vi "Generate Border User Layer.vi"(10 "color(black)":u32(colorbox)) -> (3 "User Layer data":T1)   [LabVIEW 2020, in "LabVIEW Icon API.lvlib"]
doc: "Generate a default Border Image Data glyph."
uses:
  <vilib>/LabVIEW Icon API/LabVIEW Icon API.lvlib
  <vilib>/LabVIEW Icon API/API_User Layer Data.ctl
  <vilib>/Utility/miscctls.llb/LVPoint32TypeDef.ctl
  <vilib>/picture/picture.llb/imagedata.ctl
panel:
  in  "Border":string="Border"
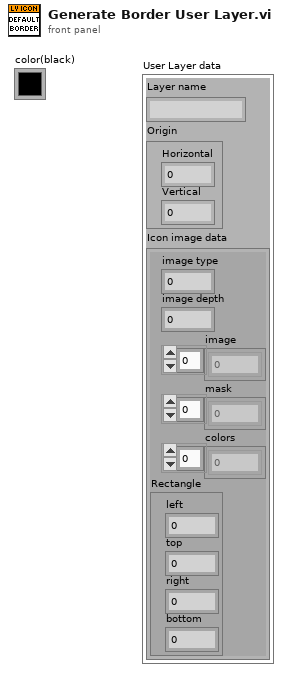
[diagram p1: front panel]
types:
  T1 = typedef "LabVIEW Icon API.lvlib/API_User Layer Data.ctl" = cluster{"Layer name":string, "Origin":T2, "Icon image data":T3}
  T2 = typedef "LVPoint32TypeDef.ctl" = cluster{"Horizontal":i32, "Vertical":i32}
  T3 = typedef "imagedata.ctl" = cluster{"image type":i32, "image depth":i32, "image":u8[], "mask":u8[], "colors":u32[], "Rectangle":cluster{"left":i16, "top":i16, "right":i16, "bottom":i16}}
  T4 = cluster{"left":i16, "top":i16, "right":i16, "bottom":i16}
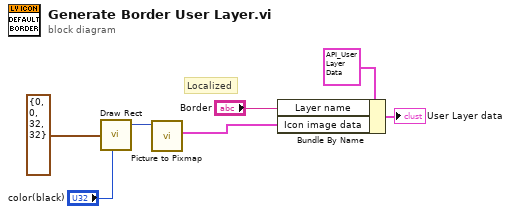
[diagram p0: block diagram]
diagram:
  # "Localized"
  n1 = call <vilib>:"Draw Rect.vi"("rect"=T4 {"left"=0, "top"=0, "right"=32, "bottom"=32}, "color(black)"="color(black)") -> ("new picture"=w2:picture)  [unwired: 7 in]
  n2 = call <vilib>:"Picture to Pixmap.vi"("picture"=w2) -> ("image data"=w1:T3)  [unwired: 9 in, 1 out]
  n3 = Bundle By Name(cluster=T1 {"Layer name"="", "Origin"={"Horizontal"=0, "Vertical"=0}, "Icon image data"={"image type"=0, "image depth"=0, "image"=[], "mask"=[], "colors"=[], "Rectangle"={"left"=0, "top"=0, "right"=0, "bottom"=0}}} ("User layer"), "Layer name"="Border", "Icon image data"=w1) -> (→"User Layer data":T1)
